vi "LymphNodeSimpleSnap.vi"() -> ()   [LabVIEW 2022 SP3]
uses:
  System.Windows.Forms
  ScanningControl/-ScanSystem/Controls/location.ctl
  ScanningControl/Motion Controllers/-MotionRoutines/MotionGlobals.vi
  Patient Routines/PatientGlobals.vi
  user32.dll
  avicap32.dll
panel:
  in  "Exit":bool
  in  "Frame to BMP":bool
  in  "PictureBox":refnum<k24>(container)
  out "Info":string
  in  "Fit Window":bool
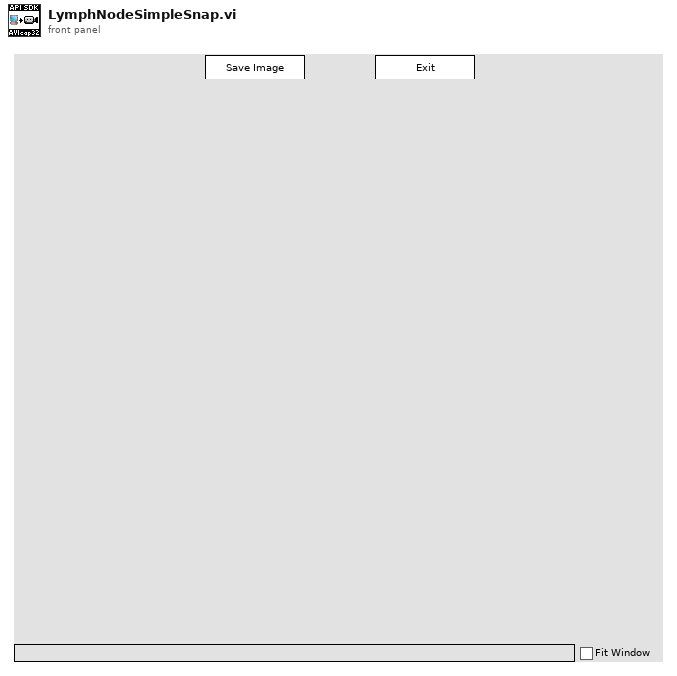
[diagram p1: front panel]
types:
  T1 = typedef "location.ctl" = enum16{"Automatic", "WCM Main", "Hawaii", "Columbia MM3000", "Columbia  NI System", "NYU", "RRI 2", "UHI Allen", "CUMC RT", "Chiba", "Stony Brook", "WCM Microscopy", "WCM Aeoretch", "WCM Optics Lab", "WCM Main 2Axis", "WCM Rotation", "WCM SAM SMAC", "SERI GP"}
  T2 = cluster{"biSize":i32, "biWidth":i32, "biHeight":i32, "biPlanes":i16, "biBitCount":i16, "biCompression":i32, "biSizeImage":i32, "biXPelsPerMeter":i32, "biYPelsPerMeter":i32, "biClrUsed":i32, "biClrImportant":i32, "Colors":u32[]}
  T3 = cluster{"uiImageWidth":u32, "uiImageHeight":u32, "fLiveWindow":u32, "fOverlayWindow":u32, "fScale":u32, "ptScroll":cluster{"x":i32, "y":i32}, "fUsingDefaultPalette":u32, "fAudioHardware":u32, "fCapFileExists":u32, "dwCurrentVideoFrame":u32, "dwCurrentVideoFramesDropped":u32, "dwCurrentWaveSamples":u32, "dwCurrentTimeElapsedMS":u32, "hPalCurrent":u32, "fCapturingNow":u32, "dwReturn":u32, "wNumVideoAllocated":u32, "wNumAudioAllocated":u32}
  T4 = cluster{"Timeout":i32, "Error":errorcluster, "hwnd":u32, "WM_CAP_START":u32, "CAPSTATUS":cluster{"uiImageWidth":u32, "uiImageHeight":u32, "fLiveWindow":u32, "fOverlayWindow":u32, "fScale":u32, "ptScroll":cluster{"x":i32, "y":i32}, "fUsingDefaultPalette":u32, "fAudioHardware":u32, "fCapFileExists":u32, "dwCurrentVideoFrame":u32, "dwCurrentVideoFramesDropped":u32, "dwCurrentWaveSamples":u32, "dwCurrentTimeElapsedMS":u32, "hPalCurrent":u32, "fCapturingNow":u32, "dwReturn":u32, "wNumVideoAllocated":u32, "wNumAudioAllocated":u32}, "BITMAPINFO":cluster{"biSize":i32, "biWidth":i32, "biHeight":i32, "biPlanes":i16, "biBitCount":i16, "biCompression":i32, "biSizeImage":i32, "biXPelsPerMeter":i32, "biYPelsPerMeter":i32, "biClrUsed":i32, "biClrImportant":i32, "Colors":u32[]}, "Preview FPS":dbl, "Capture FPS":dbl, "Camera":string}
  T5 = typedef "sizeaction.ctl" = enum32{"Minimized", "Maximized", "Resized"}
  T6 = typedef "LVRectTypeDef.ctl" = cluster{"Left":i16, "Top":i16, "Right":i16, "Bottom":i16}
  T7 = cluster{"wDeviceIndex":u32, "fHasOverlay":u32, "fHasDlgVideoSource":u32, "fHasDlgVideoFormat":u32, "fHasDlgVideoDisplay":u32, "fCaptureInitialized":u32, "fDriverSuppliesPalettes":u32, "hVideoIn":u32, "hVideoOut":u32, "hVideoExtIn":u32, "hVideoExtOut":u32}
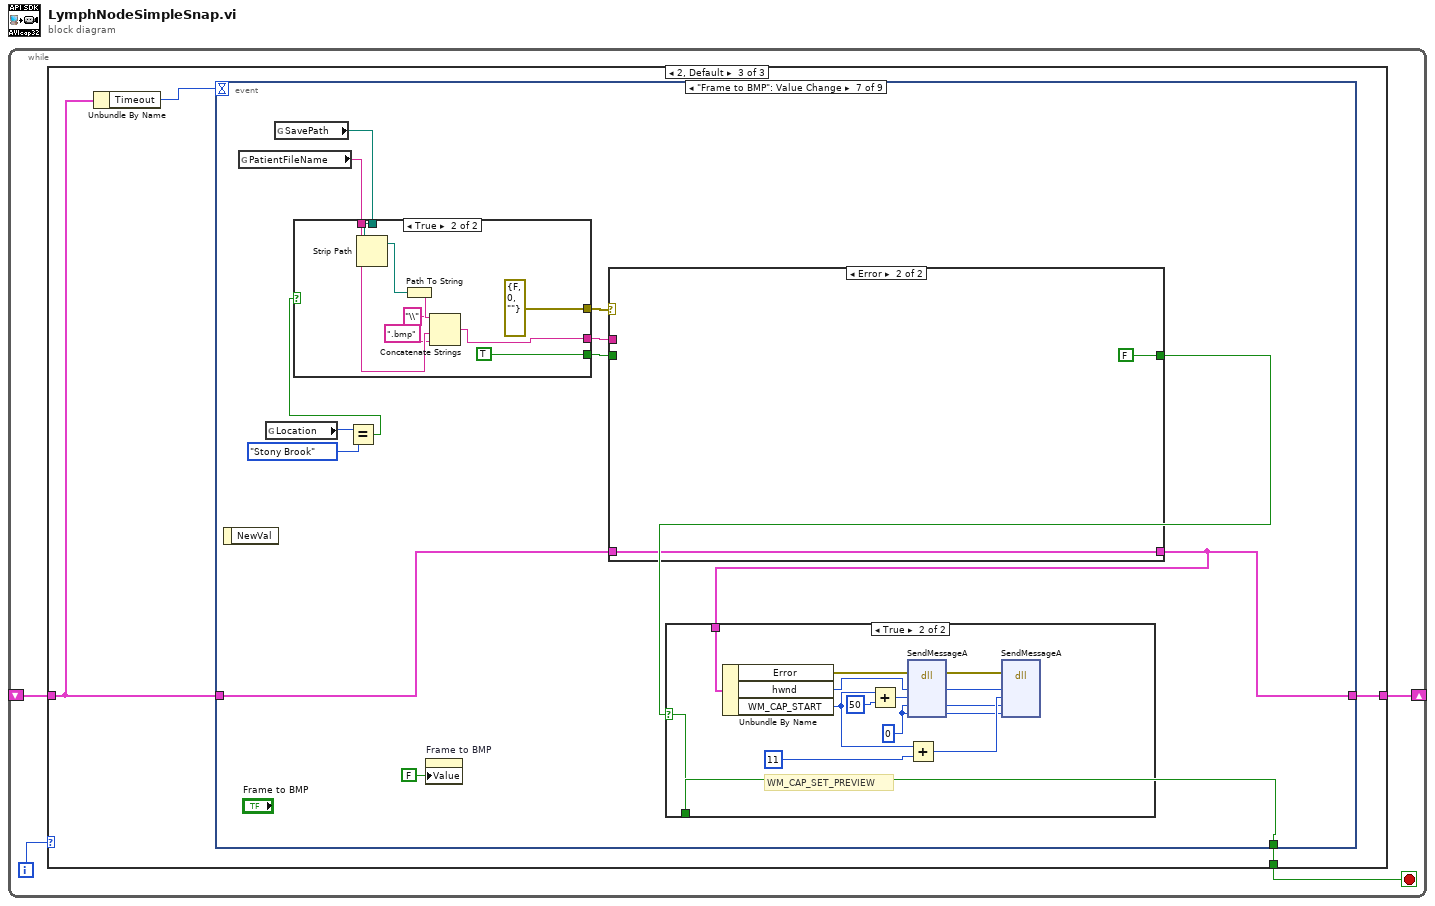
[diagram p0: block diagram]
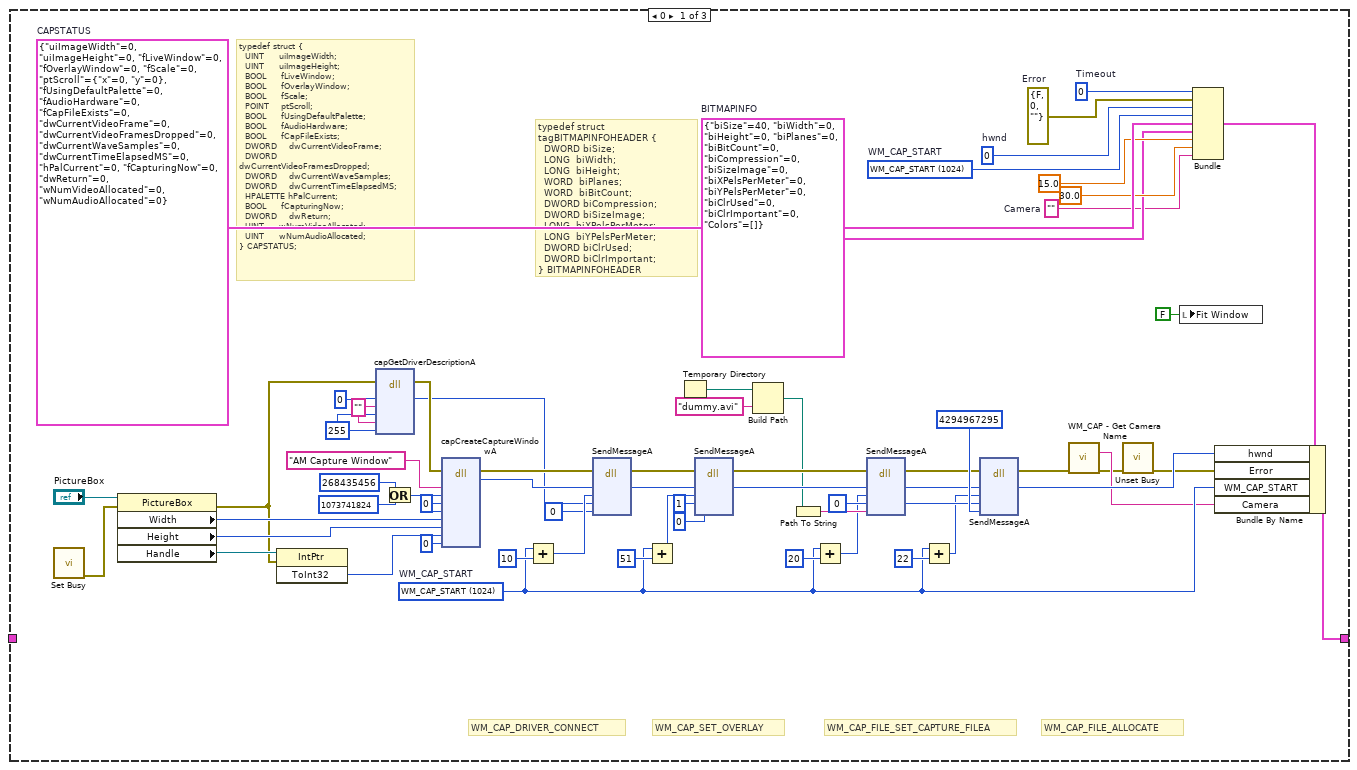
[diagram p2: hidden frame]
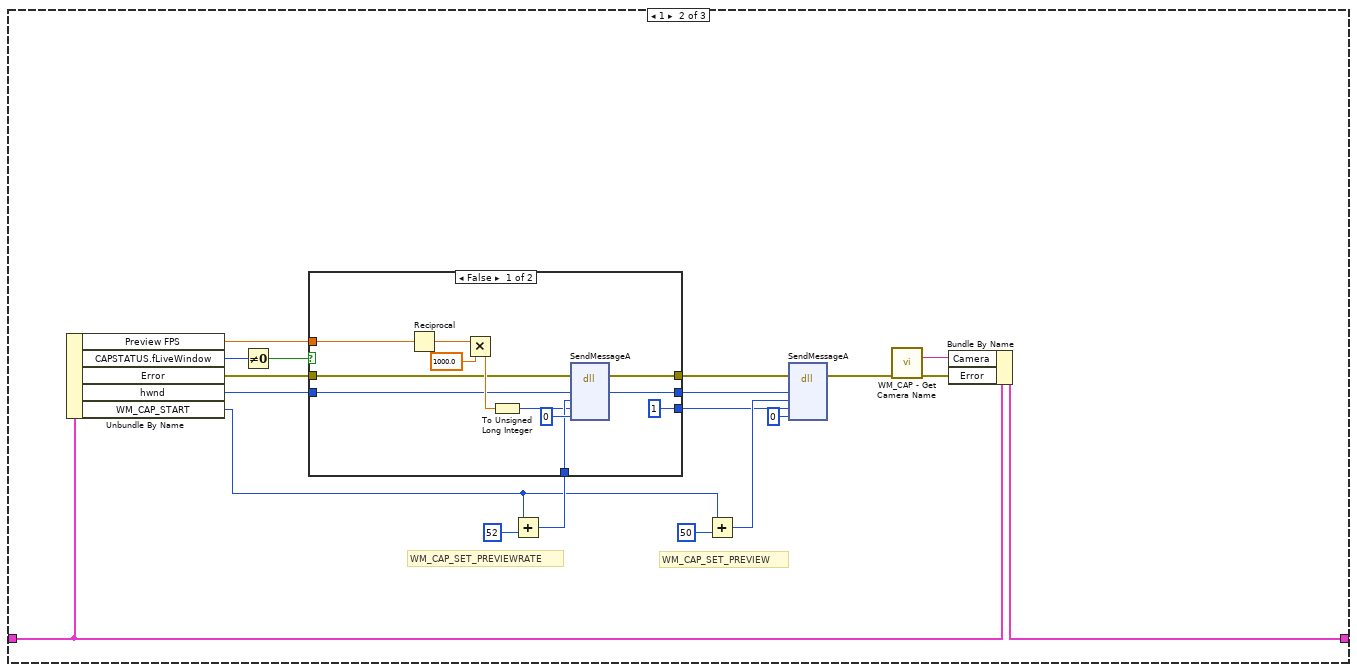
[diagram p3: hidden frame]
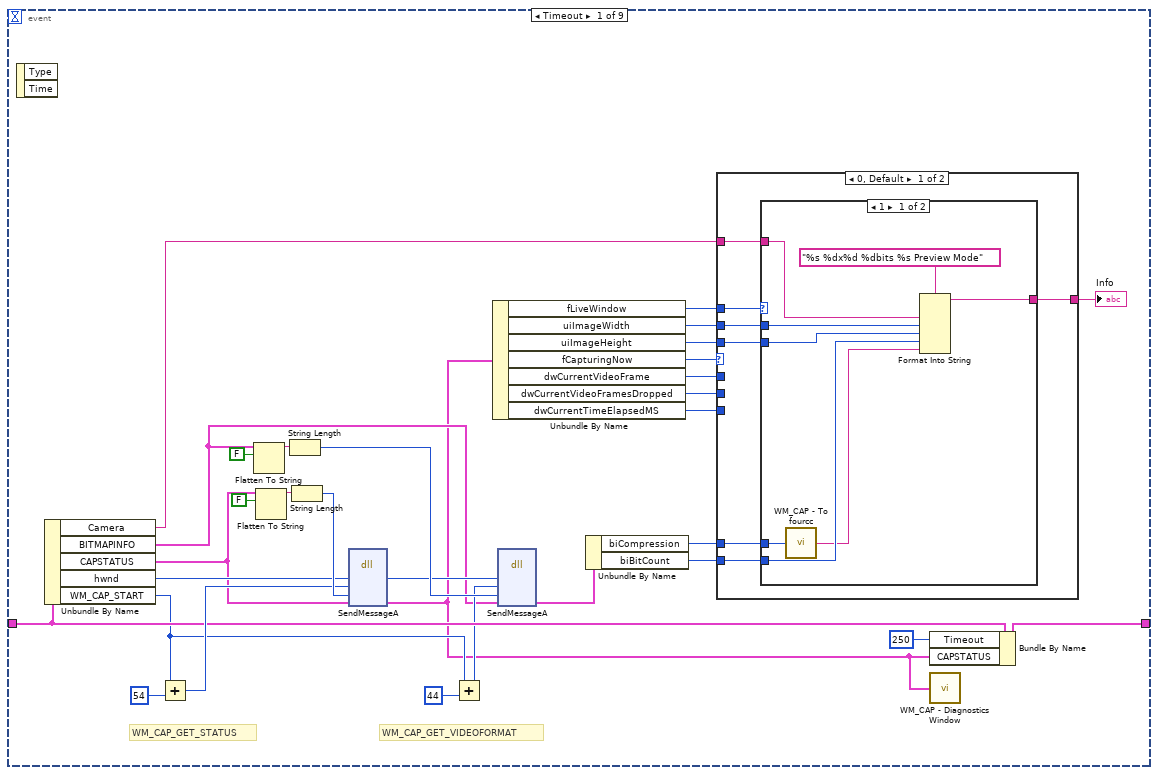
[diagram p5: hidden frame]
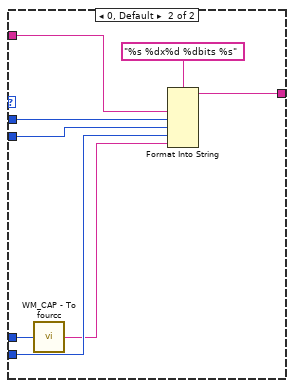
[diagram p6: hidden frame]
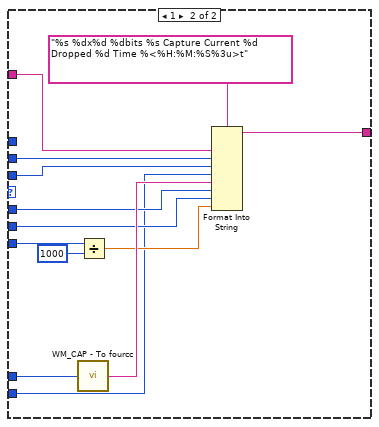
[diagram p7: hidden frame]
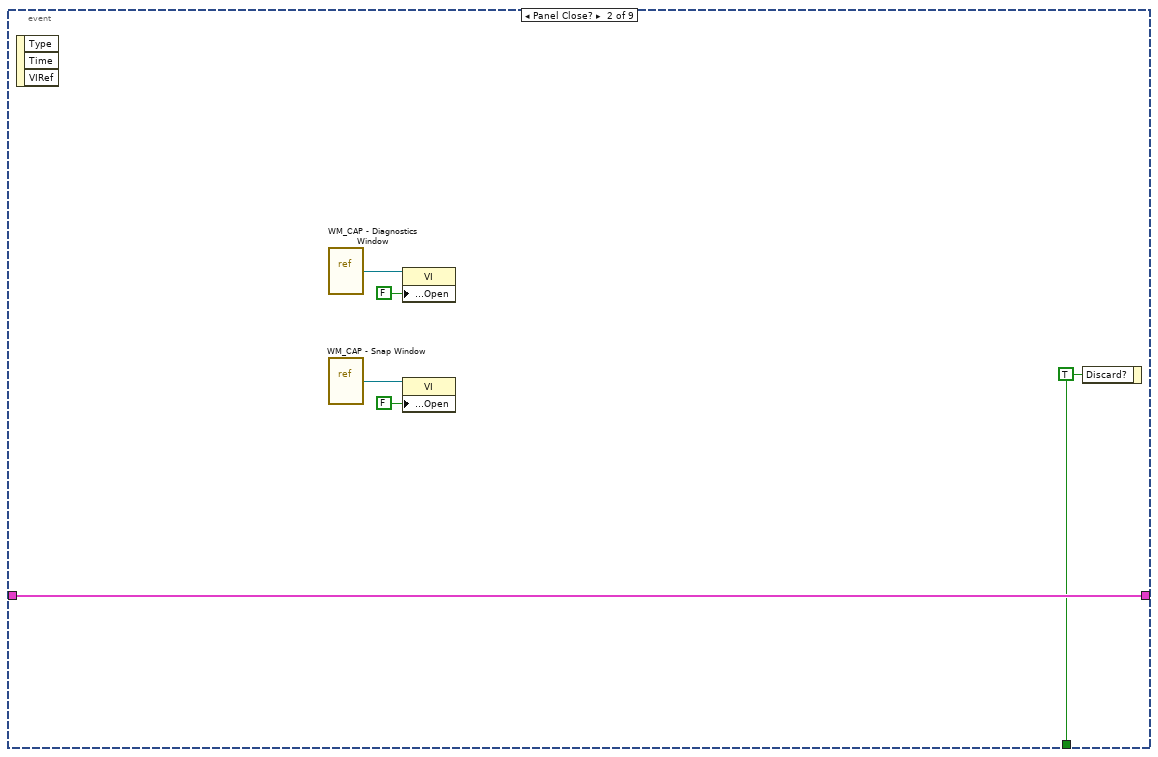
[diagram p8: hidden frame]
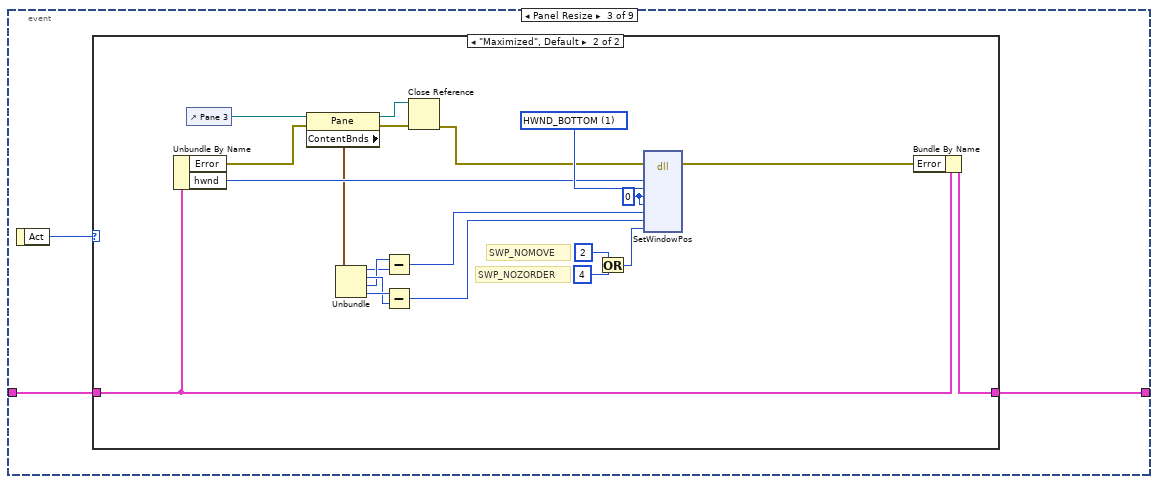
[diagram p9: hidden frame]
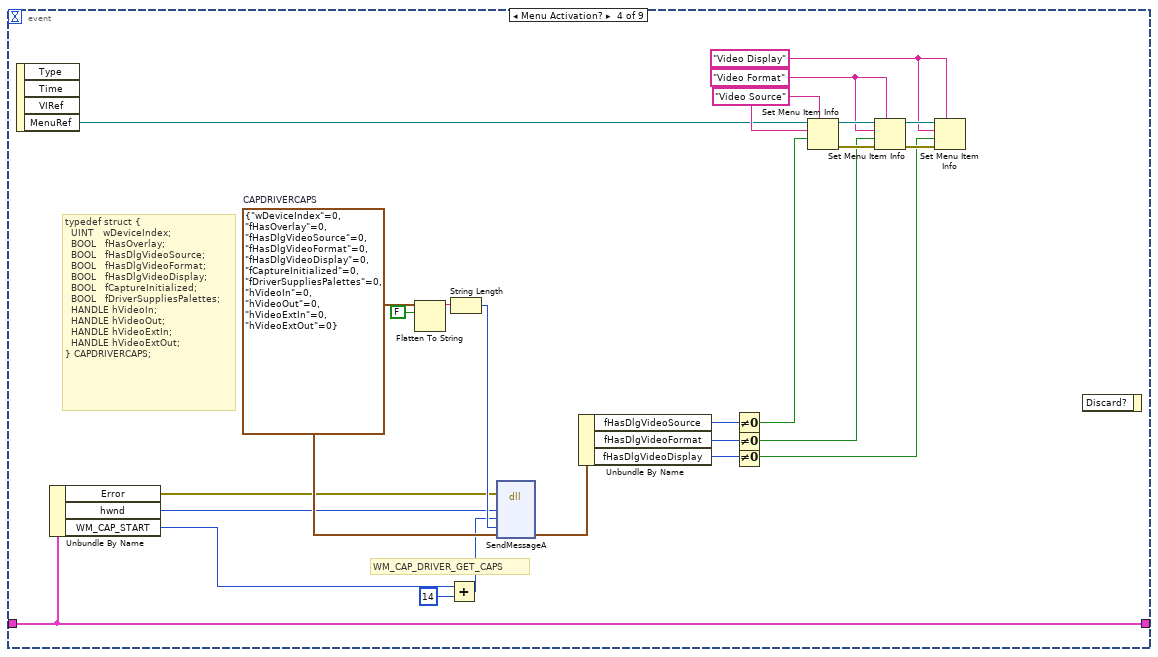
[diagram p11: hidden frame]
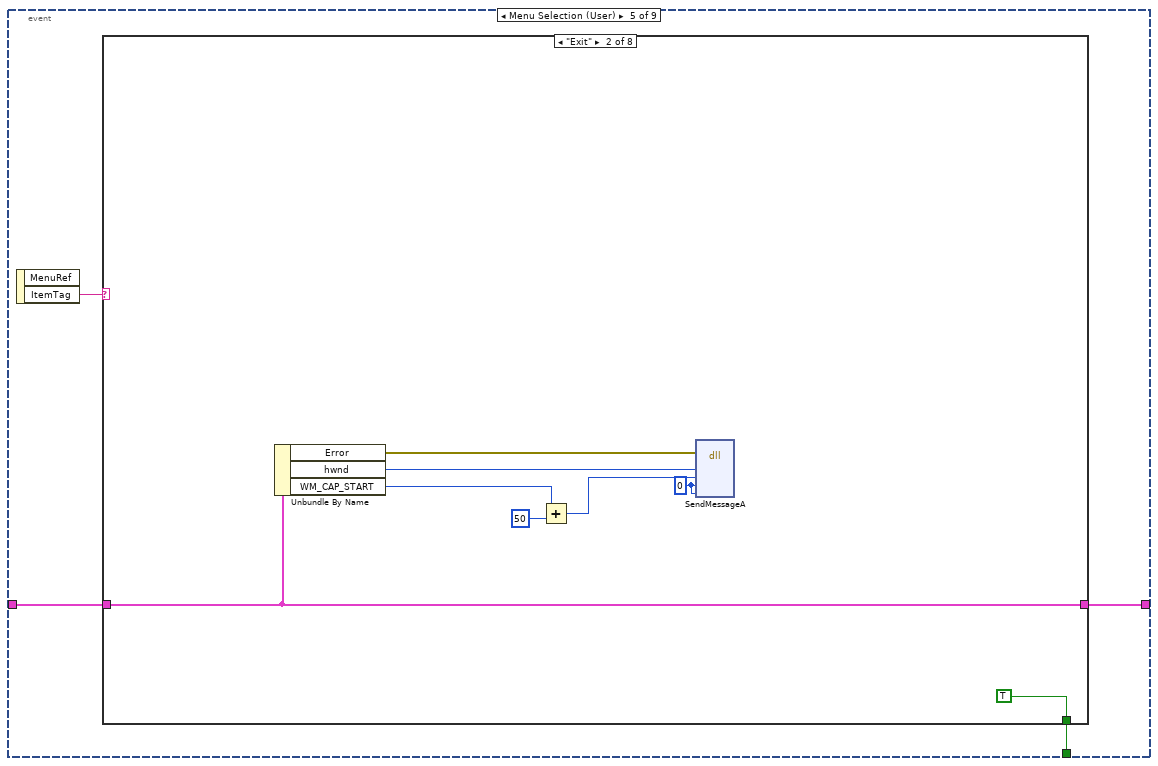
[diagram p12: hidden frame]
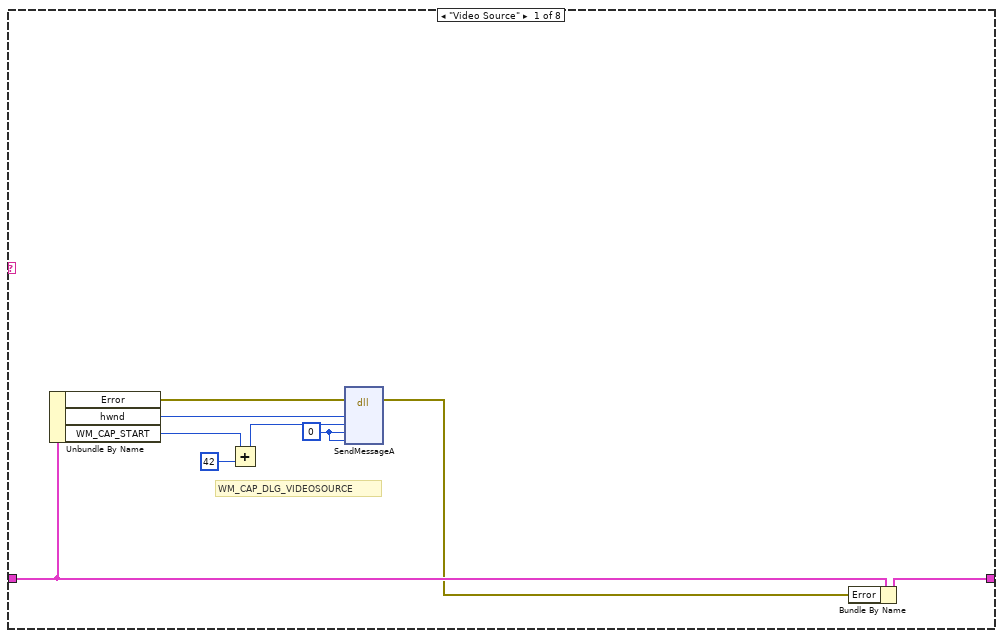
[diagram p13: hidden frame]
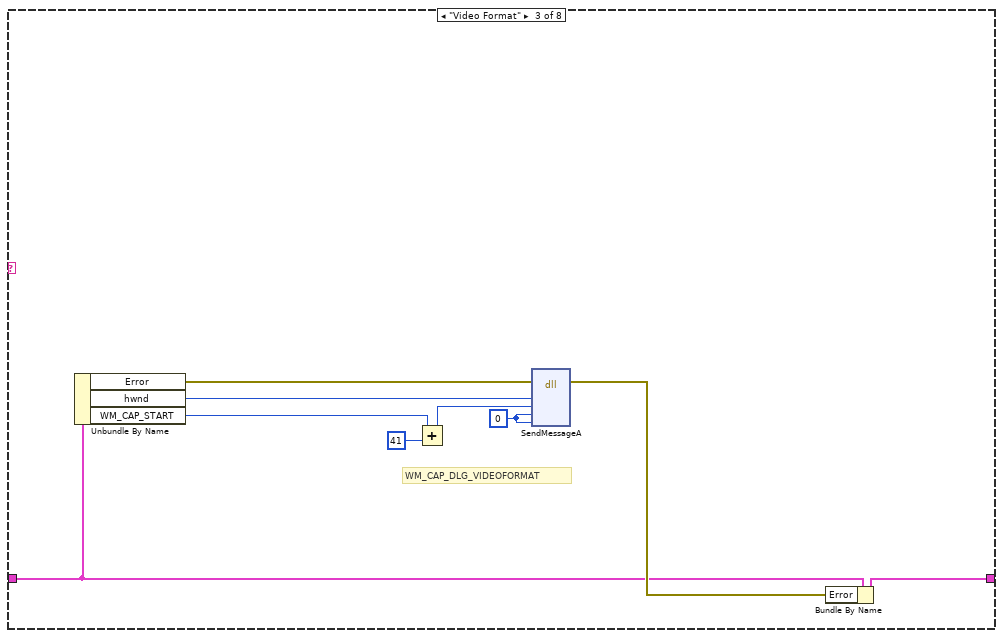
[diagram p14: hidden frame]
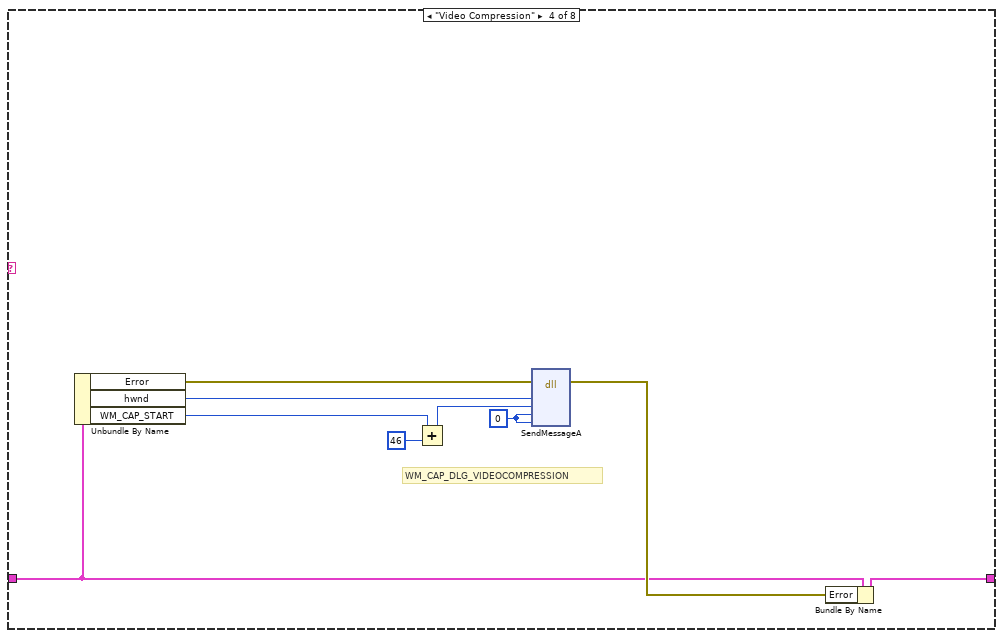
[diagram p15: hidden frame]
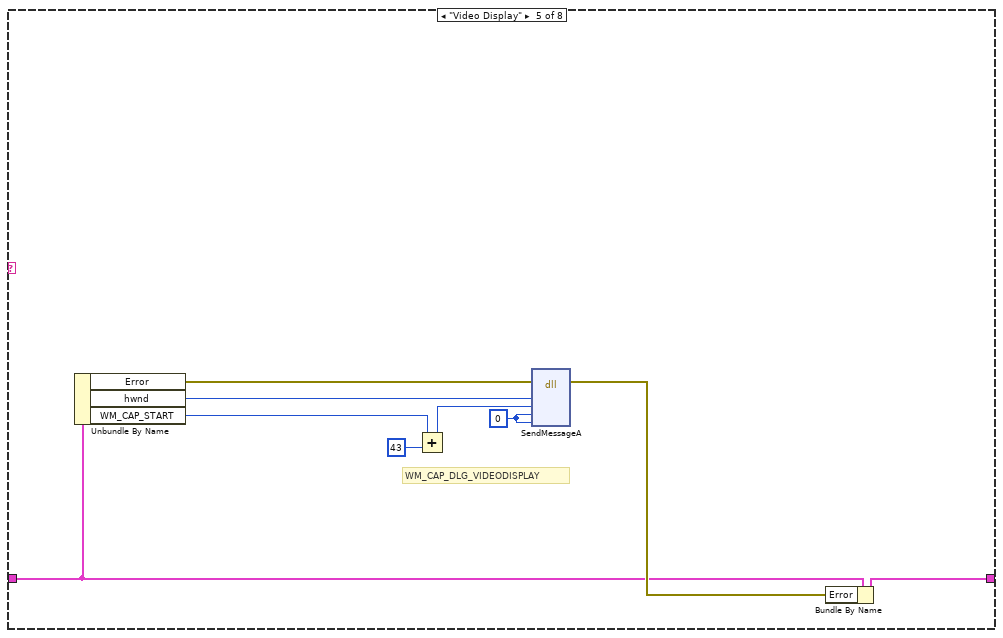
[diagram p16: hidden frame]
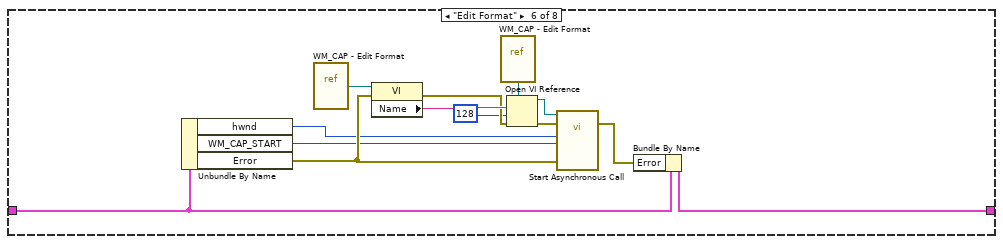
[diagram p17: hidden frame]
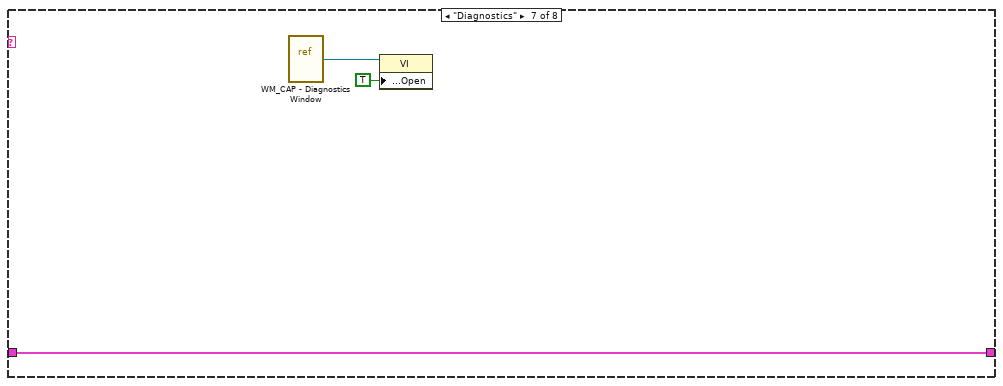
[diagram p18: hidden frame]
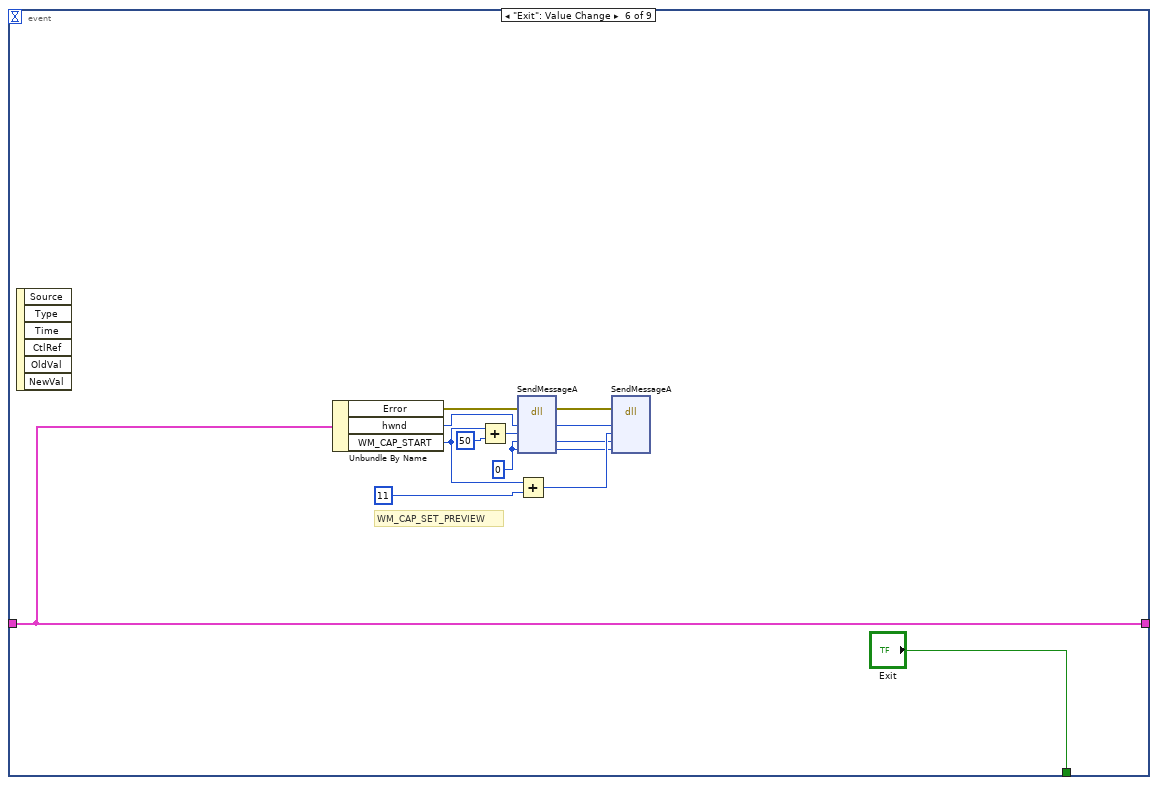
[diagram p20: hidden frame]
diagram:
  n1 = while {
    shift-right: [w3] -> _
    shift-left: _ -> [w2]
    i -> [w4]
    stop <- w1 stop-if-true
    n2 = case shown="2, Default" w4 {
      tunnel: [w47 w68 w103] -> w3
      tunnel: w2 -> [_ w67 w102]
      tunnel: [_ _ w100] -> w1
      frame 0 {
        w8 = ""  # Camera
        w12 = T2 {"biSize"=40, "biWidth"=0, "biHeight"=0, "biPlanes"=0, "biBitCount"=0, "biCompression"=0, "biSizeImage"=0, "biXPelsPerMeter"=0, "biYPelsPerMeter"=0, "biClrUsed"=0, "biClrImportant"=0, "Colors"=[]}  # BITMAPINFO
        w17 = T3 {"uiImageWidth"=0, "uiImageHeight"=0, "fLiveWindow"=0, "fOverlayWindow"=0, "fScale"=0, "ptScroll"={"x"=0, "y"=0}, "fUsingDefaultPalette"=0, "fAudioHardware"=0, "fCapFileExists"=0, "dwCurrentVideoFrame"=0, "dwCurrentVideoFramesDropped"=0, "dwCurrentWaveSamples"=0, "dwCurrentTimeElapsedMS"=0, "hPalCurrent"=0, "fCapturingNow"=0, "dwReturn"=0, "wNumVideoAllocated"=0, "wNumAudioAllocated"=0}  # CAPSTATUS
        w22 = u32 1024 items=["WM_CAP_START"=1024]  # WM_CAP_START
        w23 = u32 1024 items=["WM_CAP_START"=1024]  # WM_CAP_START
        w48 = u32 0  # hwnd
        w55 = u32 0 ("x")
        w61 = 255 ("cbName")
        w62 = ""
        w65 = errorcluster {"status"=FALSE, "code"=0, "source"=""}  # Error
        w66 = 0  # Timeout
        # "typedef struct tagBITMAPINFOHEADER {\n  DWORD biSize;\n  LONG  biWidth;\n  LONG  biHeight;\n  WORD  biPlanes;\n  WORD  biBitCount;\n  DWORD biCompression;\n  DWORD biSizeImage;\n  LONG  biXPelsPerMeter;\n  LONG  biYPelsPerMeter;\n  DWORD biClrUsed;\n  DWORD biClrImportant;\n} BITMAPINFOHEADER"
        # "typedef struct {\n  UINT     uiImageWidth;\n  UINT     uiImageHeight;\n  BOOL     fLiveWindow;\n  BOOL     fOverlayWindow;\n  BOOL     fScale;\n  POINT    ptScroll;\n  BOOL     fUsingDefaultPalette;\n  BOOL     fAudioHardware;\n  BOOL     fCapFileExists;\n  DWORD    dwCurrentVideoFrame;\n  DWORD    dwCurrentVideoFramesDropped;\n  DWORD    dwCurrentWaveSamples;\n  DWORD    dwCurrentTimeElapsedMS;\n  HPALETTE hPalCurrent;\n  BOOL     fCapturingNow;\n  DWORD    dwReturn;\n  UINT     wNumVideoAllocated;\n  UINT     wNumAudioAllocated;\n} CAPSTATUS;"
        # "WM_CAP_FILE_ALLOCATE"
        # "WM_CAP_FILE_SET_CAPTURE_FILEA"
        # "WM_CAP_SET_OVERLAY"
        # "WM_CAP_DRIVER_CONNECT"
        n3 = call <vilib>:"Set Busy.vi"() -> ("error out"=w19:errorcluster)  [unwired: 10 in, 1 out]
        n4 = property class="PictureBox"(reference="PictureBox", error in=w19) -> (error out=w16:errorcluster, "Width"=w59:i32, "Height"=w60:i32, "Handle"=w57:refnum<k24>)  [unwired: 1 out]
        n5 = invoke class="IntPtr" method="ToInt32"(reference=w57, error in=w16) -> ("ToInt32"=w58:i32)  [unwired: 1 in, 2 out]
        n6 = dll-call lib="avicap32.dll" fn="capGetDriverDescriptionA"(error in=w16, "wDriverIndex"=0, "lpszName"=w62, "cbName"=w61, "lpszVer"=w62, "cbVer"=w61) -> (error out=w49:errorcluster, "wDriverIndex"=w20:i32)  [unwired: 7 in, 1 out]
        n7 = Or(x=u32 268435456, y=u32 1073741824) -> (x .or. y?=w54:u32)
        n8 = dll-call lib="avicap32.dll" fn="capCreateCaptureWindowA"(error in=w49, "lpszWindowName"="AM Capture Window", "dwStyle"=w54, "x"=w55, "y"=w55, "nWidth"=w59, "nHeight"=w60, "hwnd"=w58, "nID"=u32 0) -> (error out=w46:errorcluster, "return type"=w44:u32)  [unwired: 10 in, 1 out]
        n9 = Add(x=w23, y=u32 10) -> (x+y=w43:u32)
        n10 = dll-call lib="user32.dll" fn="SendMessageA"(error in=w46, "hwnd"=w44, "msg"=w43, "wParam"=w20, "lparam"=u32 0 ("msg")) -> (error out=w39:errorcluster, "hwnd"=w37:u32)  [unwired: 6 in, 1 out]
        n11 = Add(x=w23, y=u32 51) -> (x+y=w36:u32)
        n12 = Temporary Directory() -> (w11:path)
        n13 = dll-call lib="user32.dll" fn="SendMessageA"(error in=w39, "hwnd"=w37, "msg"=w36, "wParam"=u32 1, "lparam"=u32 0) -> (error out=w25:errorcluster, "hwnd"=w21:u32)  [unwired: 6 in, 1 out]
        n14 = Build Path(base path=w11, name or relative path="dummy.avi") -> (appended path=w9:path)
        n15 = Path To String(path=w9) -> (string=w29:string)
        n16 = Add(x=w23, y=u32 20) -> (x+y=w27:u32)
        n17 = dll-call lib="user32.dll" fn="SendMessageA"(error in=w25, "hwnd"=w21, "msg"=w27, "wParam"=u32 0 ("msg"), "lparam"=w29) -> (error out=w30:errorcluster, "hwnd"=w31:u32, "wParam"=w34:u32)  [unwired: 5 in, 1 out]
        n18 = Add(x=w23, y=u32 22) -> (x+y=w33:u32)
        n19 = dll-call lib="user32.dll" fn="SendMessageA"(error in=w30, "hwnd"=w31, "msg"=w33, "wParam"=w34, "lparam"=u32 4294967295) -> (error out=w6:errorcluster, "hwnd"=w24:u32)  [unwired: 6 in, 1 out]
        n20 = call "WM_CAP - Get Camera Name.vi"("error in (no error)"=w6) -> ("FriendlyName"=w7:string, "error out"=w5:errorcluster)  [unwired: 12 in, 1 out]
        n21 = call <vilib>:"Unset Busy.vi"("error in (no error)"=w5) -> ("error out"=w18:errorcluster)  [unwired: 10 in]
        n22 = local write "Fit Window"(FALSE ("Fit Window")) -> ()
        n23 = Bundle("Timeout"=w66, "Error"=w65, "hwnd"=w48, "WM_CAP_START"=w22, "CAPSTATUS"=w17, "BITMAPINFO"=w12, "Preview FPS"=15.0, "Capture FPS"=30.0, "Camera"=w8) -> (w64:T4)  [unwired: 1 in]
        n24 = Bundle By Name(cluster=w64, "hwnd"=w24, "Error"=w18, "WM_CAP_START"=w23, "Camera"=w7) -> (w47:T4)
      }
      frame 1 {
        # "WM_CAP_SET_PREVIEWRATE"
        # "WM_CAP_SET_PREVIEW"
        n25 = Unbundle By Name(w67) -> ("Preview FPS"=w76:dbl, "CAPSTATUS.fLiveWindow"=w74:u32, "Error"=w78:errorcluster, "hwnd"=w77:u32, "WM_CAP_START"=w75:u32)
        n26 = Not Equal To 0?(x=w74) -> (x != 0?=w72:bool)
        n27 = Add(x=w75, y=u32 52) -> (x+y=w83:u32)
        n28 = case shown="False" w72 {
          tunnel: w83 -> [w96 _]
          tunnel: [w91 w99] -> w84
          tunnel: w78 -> [w90 w99]
          tunnel: w77 -> [w89 w98]
          tunnel: [w88 w98] -> w85
          tunnel: w76 -> [w87 _]
          tunnel: [u32 1 ("wParam") _] -> w73
          frame False {
            n29 = Reciprocal(x=w87) -> (1/x=w95:dbl)
            n30 = Multiply(x=w95, y=1000.0) -> (x*y=w93:dbl)
            n31 = To Unsigned Long Integer(number=w93) -> (unsigned 32bit integer=w92:u32)
            n32 = dll-call lib="user32.dll" fn="SendMessageA"(error in=w90, "hwnd"=w89, "msg"=w96, "wParam"=w92, "lparam"=u32 0) -> (error out=w91:errorcluster, "hwnd"=w88:u32)  [unwired: 6 in, 1 out]
          }
          frame True {
          }
        }
        n33 = Add(x=w75, y=u32 50) -> (x+y=w80:u32)
        n34 = dll-call lib="user32.dll" fn="SendMessageA"(error in=w84, "hwnd"=w85, "msg"=w80, "wParam"=w73, "lparam"=u32 0) -> (error out=w71:errorcluster)  [unwired: 7 in, 1 out]
        n35 = call "WM_CAP - Get Camera Name.vi"("error in (no error)"=w71) -> ("FriendlyName"=w69:string, "error out"=w70:errorcluster)  [unwired: 12 in, 1 out]
        n36 = Bundle By Name(cluster=w67, "Camera"=w69, "Error"=w70) -> (w68:T4)
      }
      frame 2, Default {
        n37 = Unbundle By Name(w102) -> ("Timeout"=w101:i32)
        n38 = event shown="[6] \"Frame to BMP\": Value Change" {
          selector: _ -> [_ _ _ _ _ _ _ _ _]
          dyn-events: _ -> [_ _ _ _ _ _ _ _ _]
          timeout: w101 -> [_ _ _ _ _ _ _ _ _]
          tunnel: [w134 w176 w178 w217 w229 w297 w309 w367 w374] -> w103
          tunnel: w102 -> [w127 w176 w179 w217 w228 w297 w318 w367 w374]
          tunnel: [_ w175 _ _ w227 "Exit" w307 _ _] -> w100
          event Timeout {
            # "WM_CAP_GET_VIDEOFORMAT"
            # "WM_CAP_GET_STATUS"
            n39 = event-data() -> ()  [unwired: 1 in, 2 out]
            n40 = Unbundle By Name(w127) -> ("Camera"=w104:string, "BITMAPINFO"=w114:T2, "CAPSTATUS"=w125:T3, "hwnd"=w126:u32, "WM_CAP_START"=w115:u32)
            n41 = Add(x=w115, y=u32 54) -> (x+y=w129:u32)
            n42 = Flatten To String(anything=w114, prepend array or string size? (T)=FALSE) -> (data string=w120:string)  [unwired: 2 in, 2 out]
            n43 = Flatten To String(anything=w125, prepend array or string size? (T)=FALSE) -> (data string=w130:string)  [unwired: 2 in, 2 out]
            n44 = String Length(string=w120) -> (length=w118:i32)
            n45 = String Length(string=w130) -> (length=w132:i32)
            n46 = dll-call lib="user32.dll" fn="SendMessageA"("hwnd"=w126, "msg"=w129, "wParam"=w132, w125) -> ("hwnd"=w116:u32, w113:T3)  [unwired: 6 in, 2 out]
            n47 = Add(x=w115, y=u16 44) -> (x+y=w117:u32)
            n48 = Unbundle By Name(w113) -> ("fLiveWindow"=w108:u32, "uiImageWidth"=w123:u32, "uiImageHeight"=w122:u32, "fCapturingNow"=w124:u32, "dwCurrentVideoFrame"=w107:u32, "dwCurrentVideoFramesDropped"=w106:u32, "dwCurrentTimeElapsedMS"=w105:u32)
            n49 = dll-call lib="user32.dll" fn="SendMessageA"("hwnd"=w116, "msg"=w117, "wParam"=w118, "lparam"=w114) -> ("lparam"=w112:T2)  [unwired: 7 in, 2 out]
            n50 = Unbundle By Name(w112) -> ("biCompression"=w111:i32, "biBitCount"=w110:i16)
            n51 = case shown="0, Default" w124 {
              tunnel: w123 -> [w141 w164]
              tunnel: w122 -> [w140 w163]
              tunnel: w111 -> [w138 w170]
              tunnel: w110 -> [w139 w158]
              tunnel: [w137 w169] -> w109
              tunnel: w108 -> [w136 _]
              tunnel: w107 -> [_ w159]
              tunnel: w106 -> [_ w160]
              tunnel: w105 -> [_ w167]
              tunnel: w104 -> [w135 w165]
              frame 0, Default {
                n52 = case shown="1" w136 {
                  tunnel: w141 -> [w145 w153]
                  tunnel: w140 -> [w144 w152]
                  tunnel: w139 -> [w143 w151]
                  tunnel: w138 -> [w148 w156]
                  tunnel: [w147 w155] -> w137
                  tunnel: w135 -> [w146 w154]
                  frame 1 {
                    n53 = call "WM_CAP - To fourcc.vi"("biCompression"=w148) -> ("FOURCC"=w142:string)  [unwired: 14 in]
                    n54 = Format Into String(format string="%s %dx%d %dbits %s Preview Mode", w146, w145, w144, w143, w142) -> (resulting string=w147:string)  [unwired: 2 in, 1 out]
                  }
                  frame 0, Default {
                    n55 = call "WM_CAP - To fourcc.vi"("biCompression"=w156) -> ("FOURCC"=w150:string)  [unwired: 14 in]
                    n56 = Format Into String(format string="%s %dx%d %dbits %s", w154, w153, w152, w151, w150) -> (resulting string=w155:string)  [unwired: 2 in, 1 out]
                  }
                }
              }
              frame 1 {
                n57 = call "WM_CAP - To fourcc.vi"("biCompression"=w170) -> ("FOURCC"=w162:string)  [unwired: 14 in]
                n58 = Divide(x=w167, y=u32 1000) -> (x/y=w161:dbl)
                n59 = Format Into String(format string="%s %dx%d %dbits %s Capture Current %d Dropped %d Time %<%H:%M:%S%3u>t", w165, w164, w163, w158, w162, w159, w160, w161) -> (resulting string=w169:string)  [unwired: 2 in, 1 out]
              }
            }
            "Info" <- w109
            n60 = Bundle By Name(cluster=w127, "Timeout"=250, "CAPSTATUS"=w113) -> (w134:T4)
            n61 = call "WM_CAP - Diagnostics Window.vi"("CAPSTATUS In"=w113) -> ()  [unwired: 15 in]
          }
          event Panel Close? {
            w175 = TRUE ("Discard?")
            n62 = event-data() -> ()  [unwired: 1 in, 3 out]
            n63 = vi-ref "WM_CAP - Diagnostics Window.vi"() -> (w174:refnum<vi>)
            n64 = vi-ref "WM_CAP - Snap Window.vi"() -> (w171:refnum<vi>)
            n65 = property class="VI"(reference=w174, "Front Panel.Open"=FALSE ("Front Panel Window:Open")) -> ()  [unwired: 1 in, 2 out]
            n66 = property class="VI"(reference=w171, "Front Panel.Open"=FALSE ("Front Panel Window:Open")) -> ()  [unwired: 1 in, 2 out]
            n67 = event-data("Discard?"=w175) -> ()  [unwired: 1 in, 1 out]
          }
          event Panel Resize {
            n68 = event-data() -> ("Act"=w177:T5)  [unwired: 1 in]
            n69 = case shown="\"Maximized\", Default" w177 {
              tunnel: w179 -> [w180 w197]
              tunnel: [w180 w195] -> w178
              frame "Minimized" {
              }
              frame "Maximized", Default {
                w184 = u32 0 ("x")
                w200 = 1 items=["HWND_BOTTOM"=1, "HWND_NOTOPMOST"=-2, "HWND_TOP"=0, "HWND_TOPMOST"=-1] ("hwndInsertAfter")
                # "SWP_NOMOVE"
                # "SWP_NOZORDER"
                n70 = Unbundle By Name(w197) -> ("Error"=w188:errorcluster, "hwnd"=w196:u32)
                n71 = control-ref of="Pane 3"() -> (w181:refnum<vi>)
                n72 = property class="Pane"(reference=w181, error in=w188) -> (reference out=w187:refnum<vi>, error out=w186:errorcluster, "ContentBnds"=w193:T6)
                n73 = Unbundle(w193) -> ("Left"=w189:i16, "Top"=w191:i16, "Right"=w190:i16, "Bottom"=w192:i16)
                n74 = Subtract(x=w190, y=w189) -> (x-y=w183:i16)
                n75 = Subtract(x=w192, y=w191) -> (x-y=w182:i16)
                n76 = Close Reference(reference=w187, error in (no error)=w186) -> (error out=w185:errorcluster)
                n77 = Or(x=u32 2, y=u32 4) -> (x .or. y?=w201:u32)
                n78 = dll-call lib="user32.dll" fn="SetWindowPos"(error in=w185, "hwnd"=w196, "hwndInsertAfter"=w200, "x"=w184, "y"=w184, "cx"=w183, "cy"=w182, "uFlags"=w201) -> (error out=w194:errorcluster)  [unwired: 10 in, 1 out]
                n79 = Bundle By Name(cluster=w197, "Error"=w194) -> (w195:T4)
              }
            }
          }
          event Menu Activation? {
            w209 = "Video Display" ("item tag")
            w210 = "Video Format" ("item tag")
            w211 = "Video Source" ("item tag")
            w225 = T7 {"wDeviceIndex"=0, "fHasOverlay"=0, "fHasDlgVideoSource"=0, "fHasDlgVideoFormat"=0, "fHasDlgVideoDisplay"=0, "fCaptureInitialized"=0, "fDriverSuppliesPalettes"=0, "hVideoIn"=0, "hVideoOut"=0, "hVideoExtIn"=0, "hVideoExtOut"=0}  # CAPDRIVERCAPS
            # "WM_CAP_DRIVER_GET_CAPS"
            # "typedef struct {\n  UINT   wDeviceIndex;\n  BOOL   fHasOverlay;\n  BOOL   fHasDlgVideoSource;\n  BOOL   fHasDlgVideoFormat;\n  BOOL   fHasDlgVideoDisplay;\n  BOOL   fCaptureInitialized;\n  BOOL   fDriverSuppliesPalettes;\n  HANDLE hVideoIn;\n  HANDLE hVideoOut;\n  HANDLE hVideoExtIn;\n  HANDLE hVideoExtOut;\n} CAPDRIVERCAPS;"
            n80 = event-data() -> ("MenuRef"=w202:refnum<k9>)  [unwired: 1 in, 3 out]
            n81 = Unbundle By Name(w217) -> ("Error"=w220:errorcluster, "hwnd"=w219:u32, "WM_CAP_START"=w218:u32)
            n82 = Flatten To String(anything=w225, prepend array or string size? (T)=FALSE) -> (data string=w223:string)  [unwired: 2 in, 2 out]
            n83 = Add(x=w218, y=u32 14) -> (x+y=w222:u32)
            n84 = String Length(string=w223) -> (length=w226:i32)
            n85 = dll-call lib="user32.dll" fn="SendMessageA"(error in=w220, "hwnd"=w219, "msg"=w222, "wParam"=w226, "lparam"=w225) -> ("lparam"=w214:T7)  [unwired: 6 in, 2 out]
            n86 = Unbundle By Name(w214) -> ("fHasDlgVideoSource"=w208:u32, "fHasDlgVideoFormat"=w207:u32, "fHasDlgVideoDisplay"=w206:u32)
            n87 = Not Equal To 0?(x=w208) -> (x != 0?=w205:bool)
            n88 = Not Equal To 0?(x=w207) -> (x != 0?=w204:bool)
            n89 = Not Equal To 0?(x=w206) -> (x != 0?=w203:bool)
            n90 = Set Menu Item Info(7:w211, 9:w205, 10:w211, 11:w202) -> (0:w216:errorcluster, 3:w213:refnum<k9>)  [unwired: 3 in]
            n91 = Set Menu Item Info(7:w210, 8:w216, 9:w204, 10:w210, 11:w213) -> (0:w215:errorcluster, 3:w212:refnum<k9>)  [unwired: 2 in]
            n92 = Set Menu Item Info(7:w209, 8:w215, 9:w203, 10:w209, 11:w212) -> ()  [unwired: 2 in, 2 out]
            n93 = event-data() -> ()  [unwired: 2 in, 1 out]
          }
          event Menu Selection (User) {
            n94 = event-data() -> ("ItemTag"=w230:string)  [unwired: 1 in, 1 out]
            n95 = case shown="\"Exit\"" w230 {
              tunnel: [w234 w244 w253 w262 w271 w286 w290 w291] -> w229
              tunnel: w228 -> [w236 w244 w251 w260 w269 w287 w290 w291]
              tunnel: [_ TRUE _ _ _ _ _ _] -> w227
              frame "Video Source" {
                w239 = u32 0 ("msg")
                # "WM_CAP_DLG_VIDEOSOURCE"
                n96 = Unbundle By Name(w236) -> ("Error"=w232:errorcluster, "hwnd"=w231:u32, "WM_CAP_START"=w235:u32)
                n97 = Add(x=w235, y=u32 42) -> (x+y=w238:u32)
                n98 = dll-call lib="user32.dll" fn="SendMessageA"(error in=w232, "hwnd"=w231, "msg"=w238, "wParam"=w239, "lparam"=w239) -> (error out=w233:errorcluster)  [unwired: 7 in, 1 out]
                n99 = Bundle By Name(cluster=w236, "Error"=w233) -> (w234:T4)
              }
              frame "Exit" {
                w240 = u32 0 ("wParam")
                n100 = Unbundle By Name(w244) -> ("Error"=w243:errorcluster, "hwnd"=w242:u32, "WM_CAP_START"=w241:u32)
                n101 = Add(x=w241, y=u32 50) -> (x+y=w246:u32)
                n102 = dll-call lib="user32.dll" fn="SendMessageA"(error in=w243, "hwnd"=w242, "msg"=w246, "wParam"=w240, "lparam"=w240) -> ()  [unwired: 7 in, 2 out]
              }
              frame "Video Format" {
                w256 = u32 0 ("msg")
                # "WM_CAP_DLG_VIDEOFORMAT"
                n103 = Unbundle By Name(w251) -> ("Error"=w248:errorcluster, "hwnd"=w249:u32, "WM_CAP_START"=w250:u32)
                n104 = Add(x=w250, y=u32 41) -> (x+y=w255:u32)
                n105 = dll-call lib="user32.dll" fn="SendMessageA"(error in=w248, "hwnd"=w249, "msg"=w255, "wParam"=w256, "lparam"=w256) -> (error out=w252:errorcluster)  [unwired: 7 in, 1 out]
                n106 = Bundle By Name(cluster=w251, "Error"=w252) -> (w253:T4)
              }
              frame "Video Compression" {
                w265 = u32 0 ("msg")
                # "WM_CAP_DLG_VIDEOCOMPRESSION"
                n107 = Unbundle By Name(w260) -> ("Error"=w257:errorcluster, "hwnd"=w258:u32, "WM_CAP_START"=w259:u32)
                n108 = Add(x=w259, y=u32 46) -> (x+y=w264:u32)
                n109 = dll-call lib="user32.dll" fn="SendMessageA"(error in=w257, "hwnd"=w258, "msg"=w264, "wParam"=w265, "lparam"=w265) -> (error out=w261:errorcluster)  [unwired: 7 in, 1 out]
                n110 = Bundle By Name(cluster=w260, "Error"=w261) -> (w262:T4)
              }
              frame "Video Display" {
                w274 = u32 0 ("msg")
                # "WM_CAP_DLG_VIDEODISPLAY"
                n111 = Unbundle By Name(w269) -> ("Error"=w266:errorcluster, "hwnd"=w267:u32, "WM_CAP_START"=w268:u32)
                n112 = Add(x=w268, y=u32 43) -> (x+y=w273:u32)
                n113 = dll-call lib="user32.dll" fn="SendMessageA"(error in=w266, "hwnd"=w267, "msg"=w273, "wParam"=w274, "lparam"=w274) -> (error out=w270:errorcluster)  [unwired: 7 in, 1 out]
                n114 = Bundle By Name(cluster=w269, "Error"=w270) -> (w271:T4)
              }
              frame "Edit Format" {
                n115 = Unbundle By Name(w287) -> ("hwnd"=w276:u32, "WM_CAP_START"=w275:u32, "Error"=w277:errorcluster)
                n116 = vi-ref "WM_CAP - Edit Format.vi"() -> (w285:refnum<vi>)
                n117 = property class="VI"(reference=w285, error in=w277) -> (error out=w283:errorcluster, "Name"=w284:string)  [unwired: 1 out]
                n118 = vi-ref "WM_CAP - Edit Format.vi"() -> (w282:refnum<vi>)
                n119 = Open VI Reference(type specifier VI Refnum (for type only)=w282, vi path=w284, options=128, error in (no error)=w283) -> (vi reference=w279:refnum<vi>, error out=w280:errorcluster)  [unwired: 2 in]
                n120 = call-by-ref "Start Asynchronous Call"(reference=w279, error in=w280, "hwnd"=w276, "WM_CAP_START"=w275, "Error"=w277) -> (error out=w278:errorcluster)  [unwired: 12 in, 2 out]
                n121 = Bundle By Name(cluster=w287, "Error"=w278) -> (w286:T4)
              }
              frame "Diagnostics" {
                n122 = vi-ref "WM_CAP - Diagnostics Window.vi"() -> (w289:refnum<vi>)
                n123 = property class="VI"(reference=w289, "Front Panel.Open"=TRUE ("Front Panel Window:Open")) -> ()  [unwired: 1 in, 2 out]
              }
              frame "Error", Default {
              }
            }
          }
          event "Exit": Value Change {
            w301 = u32 0 ("wParam")
            # "WM_CAP_SET_PREVIEW"
            n124 = event-data() -> ()  [unwired: 1 in, 6 out]
            n125 = Unbundle By Name(w297) -> ("Error"=w303:errorcluster, "hwnd"=w302:u32, "WM_CAP_START"=w294:u32)
            n126 = Add(x=w294, y=u32 50) -> (x+y=w305:u32)
            n127 = dll-call lib="user32.dll" fn="SendMessageA"(error in=w303, "hwnd"=w302, "msg"=w305, "wParam"=w301, "lparam"=w301) -> (error out=w293:errorcluster, "hwnd"=w296:u32, "wParam"=w295:u32, "lparam"=w292:u32)  [unwired: 4 in, 1 out]
            n128 = Add(x=w294, y=u32 11) -> (x+y=w299:u32)
            n129 = dll-call lib="user32.dll" fn="SendMessageA"(error in=w293, "hwnd"=w296, "msg"=w299, "wParam"=w295, "lparam"=w292) -> ()  [unwired: 7 in, 2 out]
          }
          event "Frame to BMP": Value Change {
            n130 = event-data() -> ()  [unwired: 1 in, 1 out]
            n131 = global read "PatientGlobals.vi" "PatientFileName"() -> (w314:string)
            n132 = global read "MotionGlobals.vi" "Location"() -> (w313:T1)
            n133 = global read "MotionGlobals.vi" "SavePath"() -> (w315:path)
            n134 = Equal?(x=w313, y=location."Stony Brook") -> (x = y?=w311:bool)
            n135 = case shown="True" w311 {
              tunnel: [w335 w346] -> w317
              tunnel: [w343 errorcluster {"status"=FALSE, "code"=0, "source"=""} ("error out")] -> w316
              tunnel: w315 -> [w338 w351]
              tunnel: w314 -> [w337 w349]
              tunnel: [FALSE ("status") TRUE ("status")] -> w310
              frame False {
                n136 = call "File Dialog"("start path"=w338, "prompt"="Save...", "button label"="Save", "default name"=w337, "pattern (all files)"="*.bmp" ("pattern label"), "pattern label"="Bitmap Files" ("pattern (all files)")) -> ("selected path"=w336:path, "error out"=w343:errorcluster)  [unwired: 6 in, 2 out]
                n137 = Path To String(path=w336) -> (string=w335:string)
              }
              frame True {
                n138 = Strip Path(path=w351) -> (stripped path=w344:path)  [unwired: 1 out]
                n139 = Path To String(path=w344) -> (string=w350:string)
                n140 = Concatenate Strings(w350, "\\" ("string"), w349, ".bmp" ("string")) -> (w346:string)
              }
            }
            n141 = property on="Frame to BMP" class="Bool (strict)"("Value"=FALSE ("Frame to BMP")) -> ()  [unwired: 2 in, 2 out]
            n142 = case shown="Error" w316 {
              tunnel: w318 -> [w363 w365]
              tunnel: [w362 w365] -> w309
              tunnel: w317 -> [w354 _]
              tunnel: [w353 FALSE ("status")] -> w308
              tunnel: w310 -> [w353 _]
              frame No Error {
                # "WM_CAP_FILE_SAVEDIBA"
                n143 = Unbundle By Name(w363) -> ("Error"=w358:errorcluster, "hwnd"=w357:u32, "WM_CAP_START"=w356:u32)
                n144 = Add(x=w356, y=u32 25) -> (x+y=w360:u32)
                n145 = dll-call lib="user32.dll" fn="SendMessageA"(error in=w358, "hwnd"=w357, "msg"=w360, "wParam"=u32 0 ("msg"), "lparam"=w354) -> (error out=w355:errorcluster)  [unwired: 7 in, 1 out]
                n146 = Bundle By Name(cluster=w363, "Error"=w355) -> (w362:T4)
              }
              frame Error {
              }
            }
            n147 = case shown="True" w308 {
              selector: w308 -> [w319 w320]
              tunnel: w309 -> [_ w321]
              tunnel: [w319 w320] -> w307
              frame False {
              }
              frame True {
                w329 = u32 0 ("wParam")
                # "WM_CAP_SET_PREVIEW"
                n148 = Unbundle By Name(w321) -> ("Error"=w331:errorcluster, "hwnd"=w330:u32, "WM_CAP_START"=w324:u32)
                n149 = Add(x=w324, y=u32 50) -> (x+y=w333:u32)
                n150 = dll-call lib="user32.dll" fn="SendMessageA"(error in=w331, "hwnd"=w330, "msg"=w333, "wParam"=w329, "lparam"=w329) -> (error out=w323:errorcluster, "hwnd"=w326:u32, "wParam"=w325:u32, "lparam"=w322:u32)  [unwired: 4 in, 1 out]
                n151 = Add(x=w324, y=u32 11) -> (x+y=w328:u32)
                n152 = dll-call lib="user32.dll" fn="SendMessageA"(error in=w323, "hwnd"=w326, "msg"=w328, "wParam"=w325, "lparam"=w322) -> ()  [unwired: 7 in, 2 out]
              }
            }
          }
          event Key Down {
            n153 = event-data() -> ("Char"=w366:i16)  [unwired: 1 in, 9 out]
            n154 = case shown="32" w366 {
              frame 0, Default {
              }
              frame 32 {
                n155 = property on="Frame to BMP" class="Bool (strict)"("Val(Sgnl)"=TRUE ("Value (Signaling)")) -> ()  [unwired: 2 in, 2 out]
              }
            }
          }
          event "Fit Window": Value Change {
            # "WM_CAP_SET_SCALE"
            n156 = event-data() -> ()  [unwired: 1 in, 1 out]
            n157 = Unbundle By Name(w374) -> ("CAPSTATUS.fScale"=w370:u32, "Error"=w373:errorcluster, "hwnd"=w372:u32, "WM_CAP_START"=w371:u32)
            n158 = Not Equal To 0?(x=w370) -> (x != 0?=w369:bool)
            n159 = Select(t=u32 0 ("wParam"), s=w369, f=u32 1 ("wParam")) -> (s? t:f=w379:u32)
            n160 = Add(x=w371, y=u16 53) -> (x+y=w376:u32)
            n161 = dll-call lib="user32.dll" fn="SendMessageA"(error in=w373, "hwnd"=w372, "msg"=w376, "wParam"=w379, "lparam"=u32 0) -> ()  [unwired: 7 in, 2 out]
          }
        }
      }
    }
  }
